vi "Random Boolean 2.0.vi"(6 "Output Random":bool, 8 "Cycle Time":dbl, 9 "Boolean in 3":bool, 10 "Boolean in 2":bool, 11 "Boolean in 1":bool) -> (1 "Boolean out 3":bool, 2 "Boolean out 2":bool, 3 "Boolean out 1":bool)   [LabVIEW 2016]
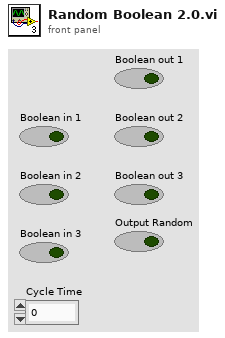
[diagram p1: front panel]
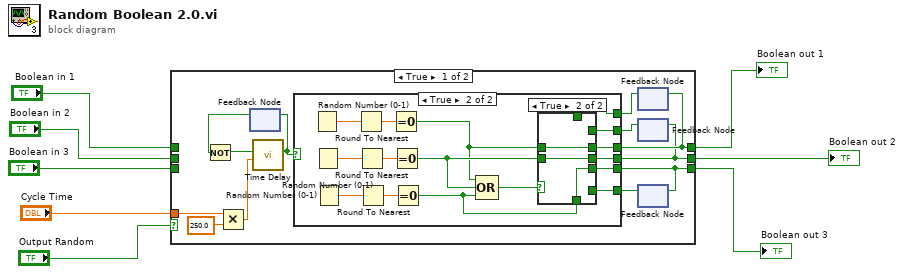
[diagram p0: block diagram]
diagram:
  n1 = case shown="True" "Output Random" {
    tunnel: [w18 w48] -> w2
    tunnel: "Boolean in 3" -> [_ w48]
    tunnel: [w19 w47] -> w4
    tunnel: "Boolean in 2" -> [_ w47]
    tunnel: "Boolean in 1" -> [_ w46]
    tunnel: [w20 w46] -> w6
    tunnel: "Cycle Time" -> [w13 _]
    frame True {
      n2 = Multiply(x=w13, y=250.0) -> (x*y=w11:dbl)
      n3 = feedback #1() -> (w14:bool)  [unwired: 1 in]
      n4 = Not(x=w14) -> (.not. x?=w10:bool)
      n5 = call "Time Delay.vi"("Time Delay"=w11, "Boolean in"=w10) -> ("Boolean out"=w9:bool)  [unwired: 9 in]
      n6 = feedback-in #1(w9) -> ()
      n7 = feedback #2() -> (w17:bool)  [unwired: 1 in]
      n8 = feedback #3() -> (w16:bool)  [unwired: 1 in]
      n9 = feedback #4() -> (w15:bool)  [unwired: 1 in]
      n10 = case shown="True" w9 {
        tunnel: [w22 w28] -> w20
        tunnel: [w21 w30] -> w19
        tunnel: [w23 w31] -> w18
        tunnel: w17 -> [w22 w24]
        tunnel: w16 -> [w21 w25]
        tunnel: w15 -> [w23 w26]
        frame False {
        }
        frame True {
          n11 = Random Number (0-1)() -> (number: 0 to 1=w39:dbl)
          n12 = Random Number (0-1)() -> (number: 0 to 1=w37:dbl)
          n13 = Random Number (0-1)() -> (number: 0 to 1=w35:dbl)
          n14 = Round To Nearest(number=w39) -> (nearest integer value=w38:dbl)
          n15 = Round To Nearest(number=w37) -> (nearest integer value=w36:dbl)
          n16 = Round To Nearest(number=w35) -> (nearest integer value=w34:dbl)
          n17 = Equal To 0?(x=w38) -> (x = 0?=w27:bool)
          n18 = Equal To 0?(x=w36) -> (x = 0?=w29:bool)
          n19 = Equal To 0?(x=w34) -> (x = 0?=w32:bool)
          n20 = Compound Arithmetic op=OR(w27, w29, w32) -> (w33:bool)
          n21 = case shown="True" w33 {
            tunnel: w32 -> [_ w45]
            tunnel: [w42 w45] -> w31
            tunnel: w29 -> [_ w44]
            tunnel: [w41 w44] -> w30
            tunnel: w27 -> [_ w43]
            tunnel: [w40 w43] -> w28
            tunnel: w26 -> [w42 _]
            tunnel: w25 -> [w41 _]
            tunnel: w24 -> [w40 _]
            frame False {
            }
            frame True {
            }
          }
        }
      }
      n22 = feedback-in #2(w20) -> ()
      n23 = feedback-in #3(w19) -> ()
      n24 = feedback-in #4(w18) -> ()
    }
    frame False {
    }
  }
  "Boolean out 1" <- w6
  "Boolean out 2" <- w4
  "Boolean out 3" <- w2
